vi "Pre Launch Init.vi"(11 "Nested in":refnum<class "Display_Console_UI.lvclass">) -> (0 "error out":errorcluster, 3 "Nested out":refnum<class "Display_Console_UI.lvclass">)   [LabVIEW 2025, in "Display_Console_UI.lvlib" / "Display_Console_UI.lvclass"]
doc: "(<B>Filename</B>: Actor Framework.lvlib:Actor.lvclass:Pre Launch Init.vi)\n\nDefines behavior that occurs after the Launch Nested Actor method is invoked but before the actor's Actor Core method begins running.\n\nBy default, this method does nothing. A descendant class may override it to define behavior."
uses:
  Display_Console_UI.lvclass
  Display_Console_UI.lvclass/Display_Console_UI.ctl
  <vilib>/ActorFramework/Actor/Actor.lvclass
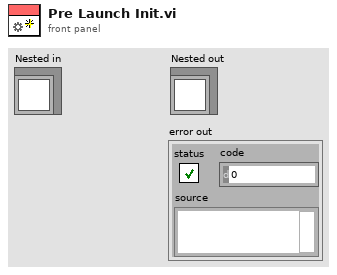
[diagram p1: front panel]
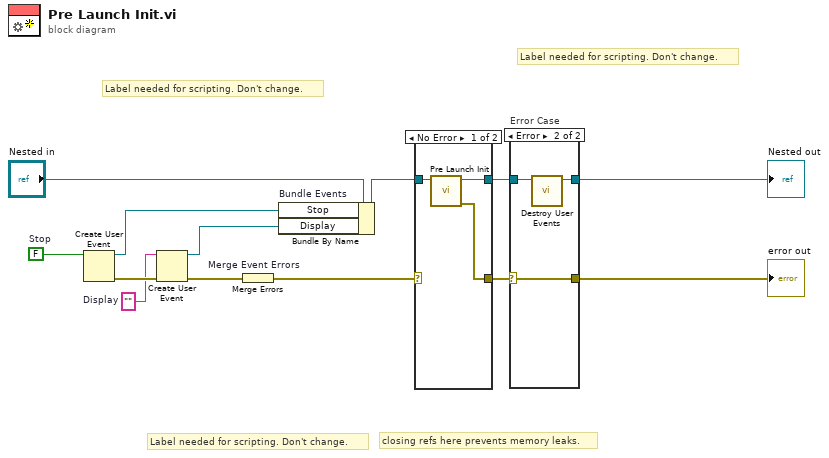
[diagram p0: block diagram]
diagram:
  w2 = ""  # Display
  w12 = FALSE  # Stop
  # "Label needed for scripting. Don't change."
  # "Label needed for scripting. Don't change."
  # "Label needed for scripting. Don't change."
  # "closing refs here prevents memory leaks."
  n1 = Create User Event(user event datatype=w12) -> (user event=w10:refnum<user-event>, error out=w4:errorcluster)  [unwired: 1 in]
  n2 = Create User Event(user event datatype=w2, error in=w4) -> (user event=w1:refnum<user-event>, error out=w3:errorcluster)
  n3 = Merge Errors "Merge Event Errors"(w3) -> (w6:errorcluster)
  n4 = Bundle By Name "Bundle Events"(cluster="Nested in", "Stop"=w10, "Display"=w1) -> (w7:refnum<class "Display_Console_UI.lvclass">)
  n5 = case shown="No Error" w6 {
    selector: w6 -> [_ w18]
    tunnel: [w16 w17] -> w8
    tunnel: w7 -> [w15 w17]
    tunnel: [w14 w18] -> w5
    frame No Error {
      n6 = call-parent "Pre Launch Init.vi"("Actor in"=w15) -> ("error out"=w14:errorcluster, "Actor out"=w16:refnum<class "Display_Console_UI.lvclass">)  [unwired: 9 in]
    }
    frame Error {
    }
  }
  n7 = case "Error Case" shown="Error" w5 {
    selector: w5 -> [w19 w23]
    tunnel: w8 -> [w20 w22]
    tunnel: [w20 w21] -> w11
    tunnel: [w19 w23] -> w9
    frame No Error {
    }
    frame Error {
      n8 = call "Destroy User Events.vi"("UI Template in"=w22) -> ("UI Template out"=w21:refnum<class "Display_Console_UI.lvclass">)  [unwired: 10 in]
    }
  }
  "error out" <- w9
  "Nested out" <- w11
